vi "Remove RTV [by name].vi"(0 "RT Variables in":refnum<class "RT Variables.lvclass">, 5 "RTV name":string, 11 "error in (no error)":errorcluster) -> (4 "RT Variables out":refnum<class "RT Variables.lvclass">, 15 "error out":errorcluster)   [LabVIEW 2019, in "LSL.lvlib" / "RT Variables.lvclass"]
uses:
  RT Variables.lvclass
  RT Variables.lvclass/RT Variables.ctl
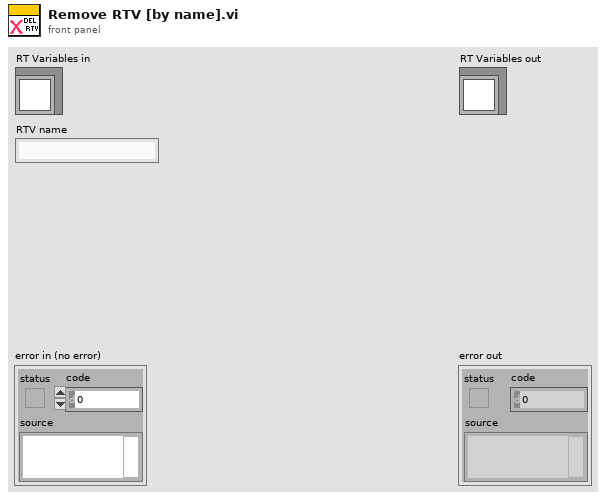
[diagram p1: front panel]
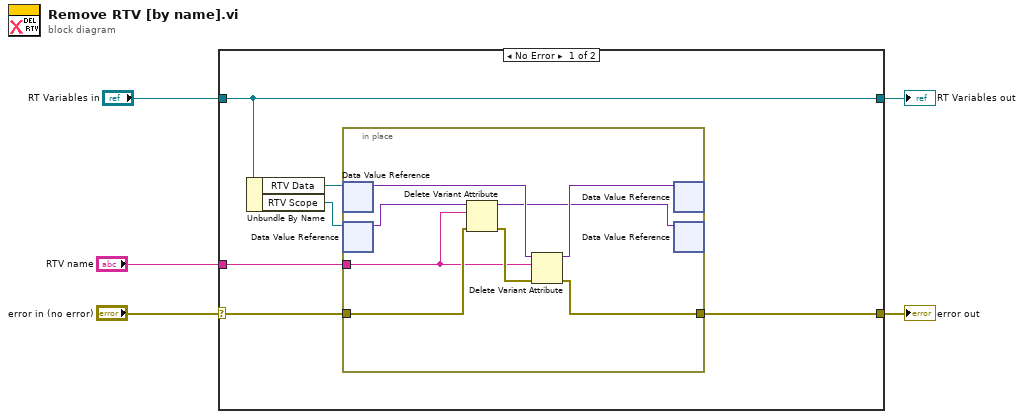
[diagram p0: block diagram]
diagram:
  n1 = case shown="No Error" "error in (no error)" {
    selector: "error in (no error)" -> [w11 w21]
    tunnel: [w10 w21] -> w4
    tunnel: "RTV name" -> [w9 _]
    tunnel: "RT Variables in" -> [w6 w20]
    tunnel: [w6 w20] -> w1
    frame No Error {
      n2 = Unbundle By Name(w6) -> ("RTV Data"=w8:refnum<data-value>, "RTV Scope"=w7:refnum<data-value>)
      n3 = in-place {
        in-place-border: w11 -> [w19]
        in-place-border: [w17] -> w10
        in-place-border: w9 -> [w16]
        n4 = in-place-dvr #1(w8) -> (w15:variant)  [unwired: 1 out]
        n5 = in-place-dvr #2(w7) -> (w12:variant)  [unwired: 1 out]
        n6 = Delete Variant Attribute(4:w19, 6:w16, 7:w12) -> (0:w18:errorcluster, 3:w13:variant)  [unwired: 1 out]
        n7 = Delete Variant Attribute(4:w18, 6:w16, 7:w15) -> (0:w17:errorcluster, 3:w14:variant)  [unwired: 1 out]
        n8 = in-place-dvr #1(w14) -> ()  [unwired: 2 out]
        n9 = in-place-dvr #2(w13) -> ()  [unwired: 2 out]
      }
    }
    frame Error {
    }
  }
  "error out" <- w4
  "RT Variables out" <- w1
